vi "Write command in.vi"(8 "error in (no error)":errorcluster, 10 "command in":T1, 11 "Motor in":refnum<class "Motor.lvclass">) -> (0 "error out":errorcluster, 3 "Motor out":refnum<class "Motor.lvclass">)   [LabVIEW 2018, in "Motor.lvclass"]
uses:
  Motor.lvclass
  Motor.lvclass/Motor.ctl
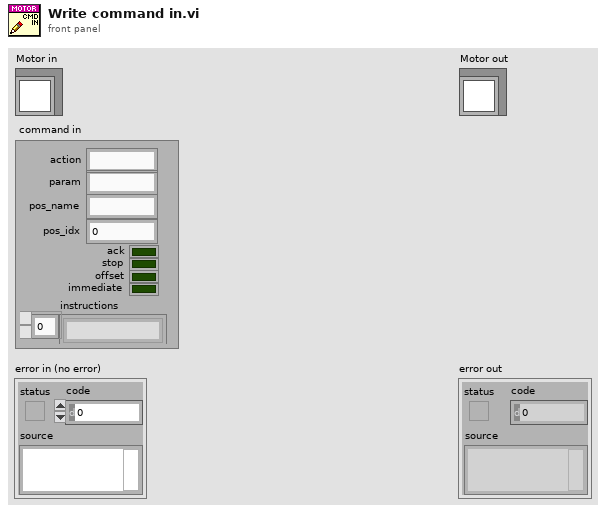
[diagram p1: front panel]
types:
  T1 = cluster{"action":string, "param":string, "pos_name":string, "pos_idx":i32, "ack":bool, "stop":bool, "offset":bool, "immediate":bool, "instructions":string[]}
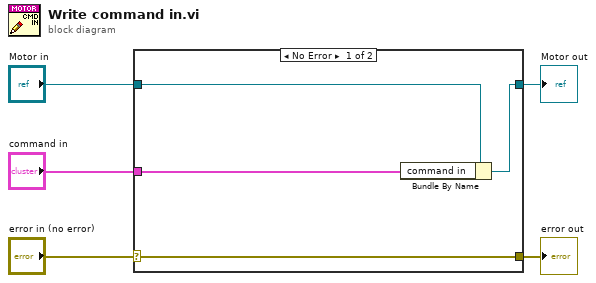
[diagram p0: block diagram]
diagram:
  n1 = case shown="No Error" "error in (no error)" {
    selector: "error in (no error)" -> [w9 w10]
    tunnel: [w9 w10] -> w4
    tunnel: [w7 w11] -> w2
    tunnel: "Motor in" -> [w8 w11]
    tunnel: "command in" -> [w6 _]
    frame No Error {
      n2 = Bundle By Name(cluster=w8, "command in"=w6) -> (w7:refnum<class "Motor.lvclass">)
    }
    frame Error {
    }
  }
  "error out" <- w4
  "Motor out" <- w2
